vi "Averages of Rows of 2D Array.vi"(11 "input array (2D)":dbl[][](array[numeric])) -> (3 "averages of rows of 2D array":dbl[](array[numeric]))   [LabVIEW 2017]
uses:
  <vilib>/Analysis/baseanly.llb/Mean (DBL).vi
  <vilib>/Analysis/NI_AALBase.lvlib
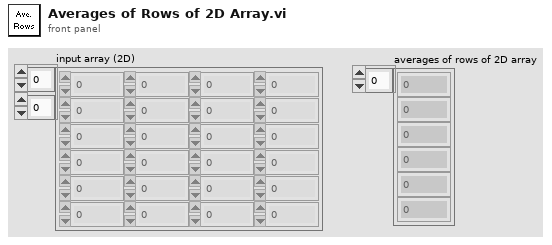
[diagram p1: front panel]
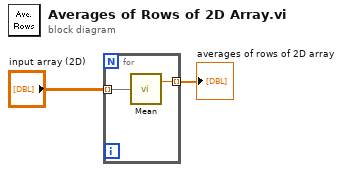
[diagram p0: block diagram]
diagram:
  n1 = for {
    tunnel: "input array (2D)" -> [w4] mode=indexing
    tunnel: [w3] -> w1 mode=indexing
    n2 = call-poly <vilib>:"Mean.vi"("X"=w4) -> ("mean"=w3:dbl)  [unwired: 1 out]
  }
  "averages of rows of 2D array" <- w1
